vi "LDA2_Safety.vi"(1 "Adam Loop Count":i32, 2 "Ch Names":string[](array[string]), 3 "Values":dbl[](array[numeric]) format="%.2f") -> (0 "Scan comment":string)   [LabVIEW 2010]
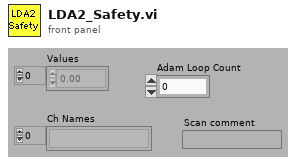
[diagram p1: front panel]
types:
  T1 = typedef "LVDateTimeRec.ctl" = cluster{"fractional second":dbl, "second":i32, "minute":i32, "hour":i32, "day of month":i32, "month":i32, "year":i32, "day of week":i32, "day of year":i32, "DST":i32}
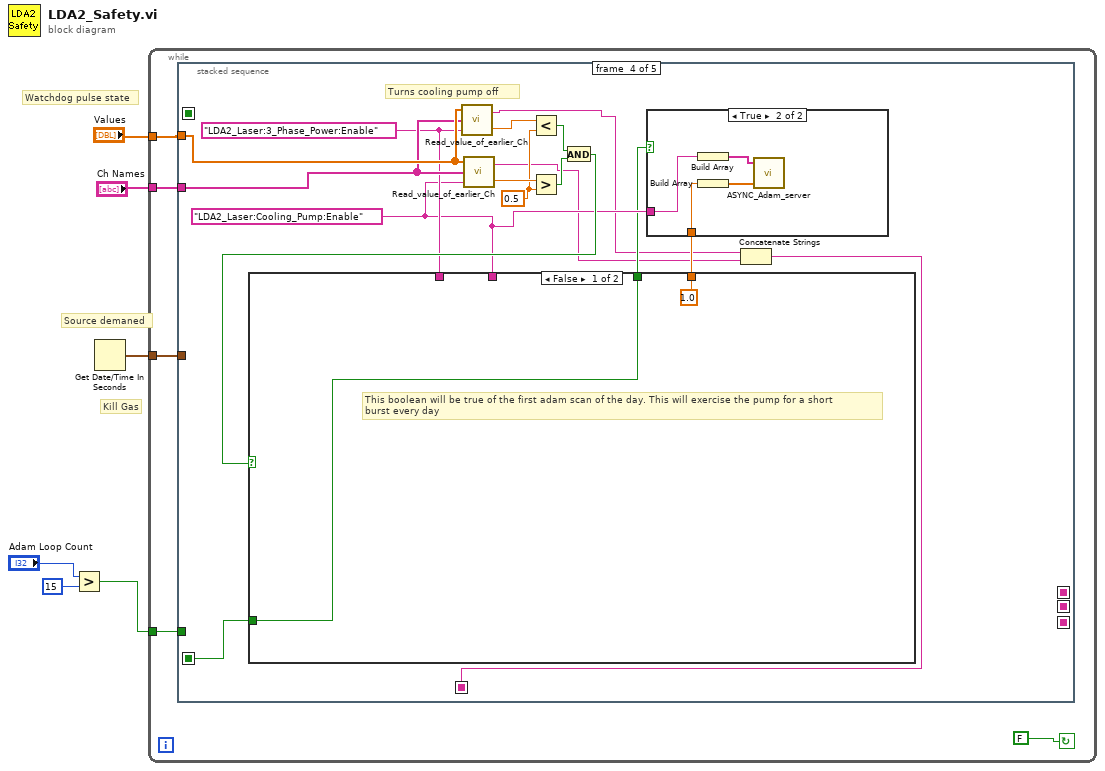
[diagram p0: block diagram]
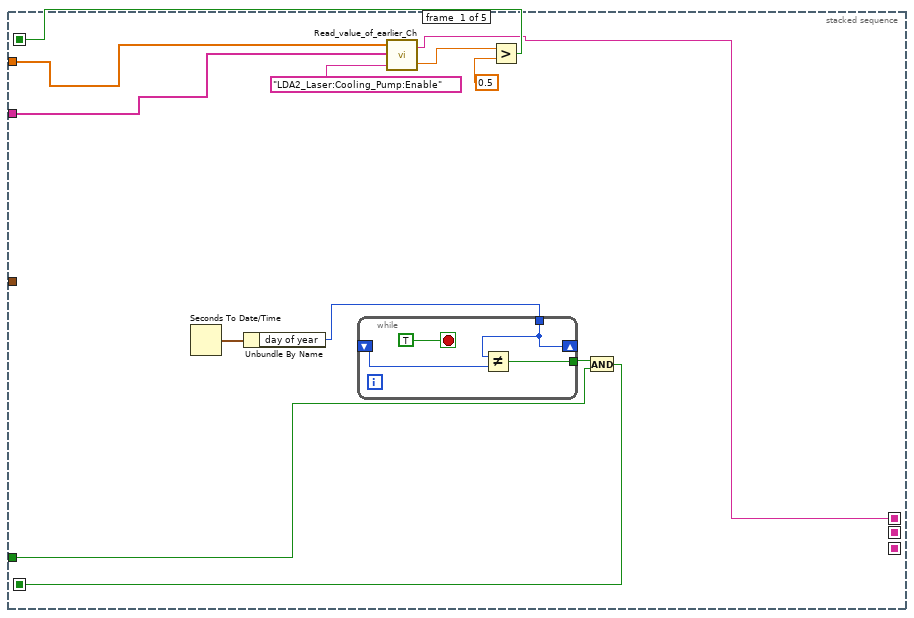
[diagram p2: hidden frame]
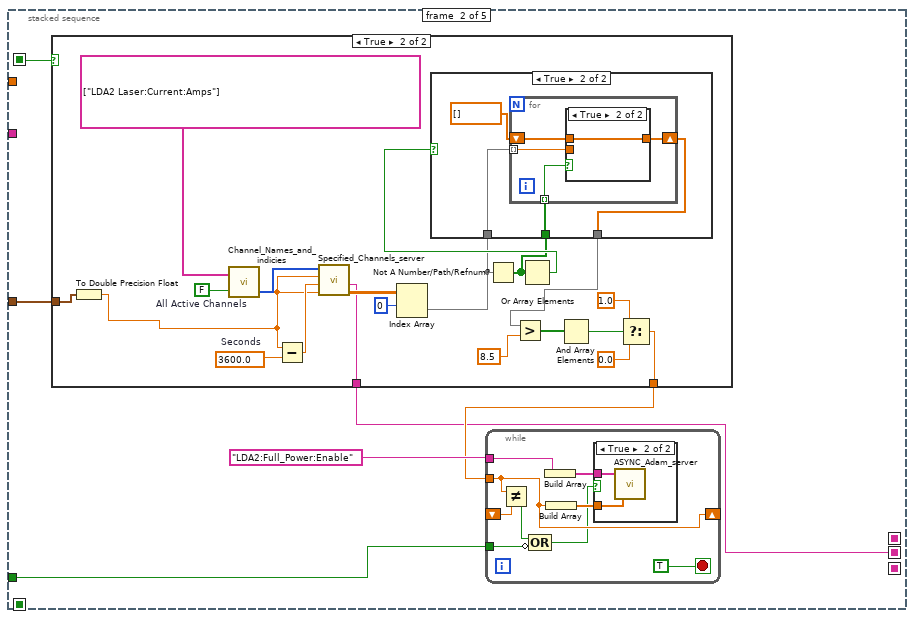
[diagram p3: hidden frame]
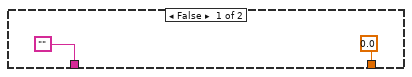
[diagram p5: hidden frame]
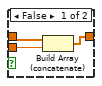
[diagram p7: hidden frame]
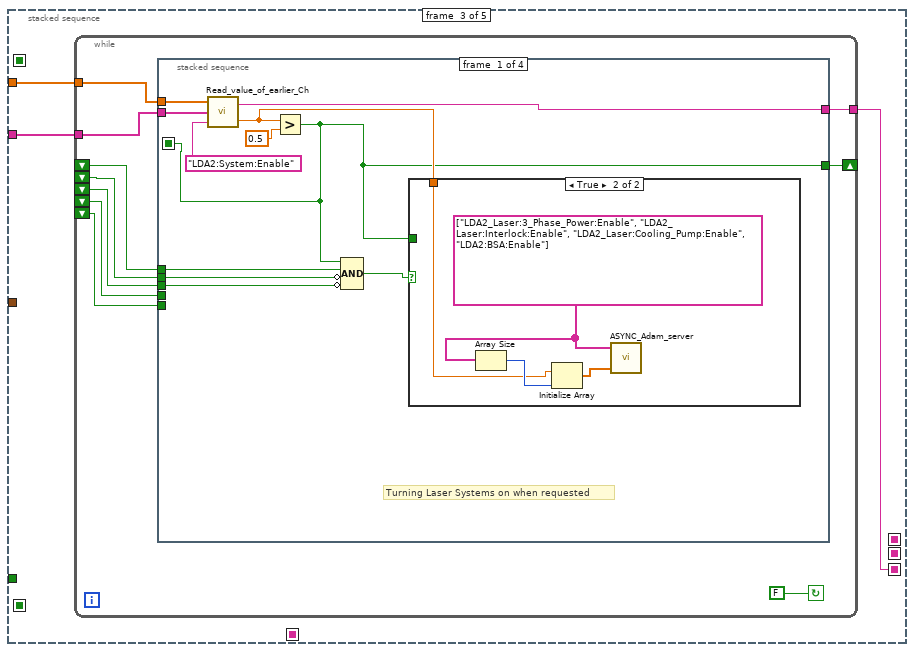
[diagram p8: hidden frame]
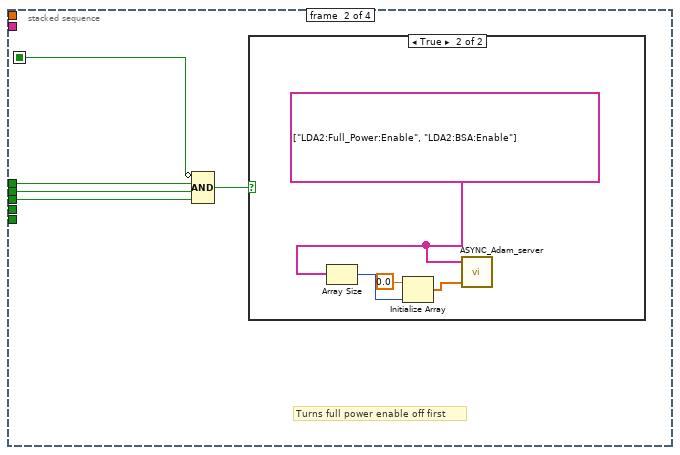
[diagram p10: hidden frame]
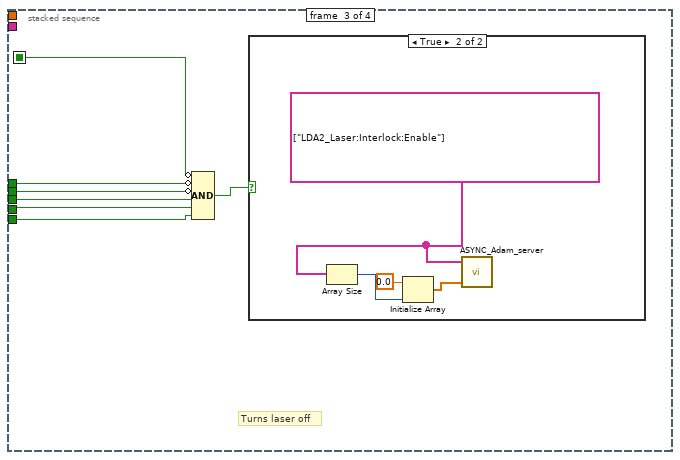
[diagram p12: hidden frame]
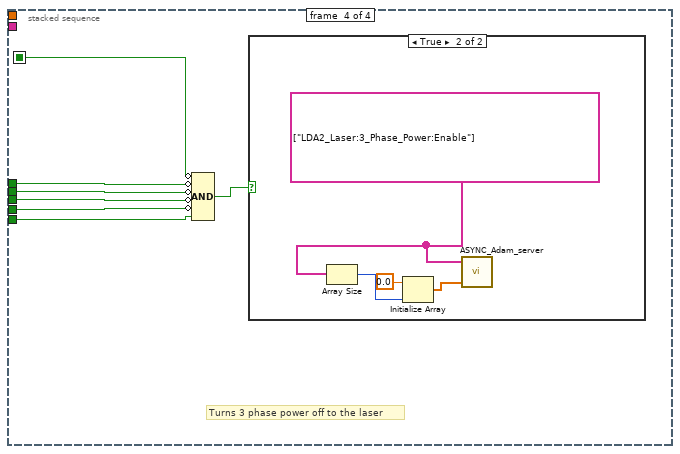
[diagram p14: hidden frame]
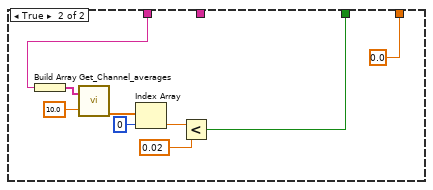
[diagram p17: hidden frame]
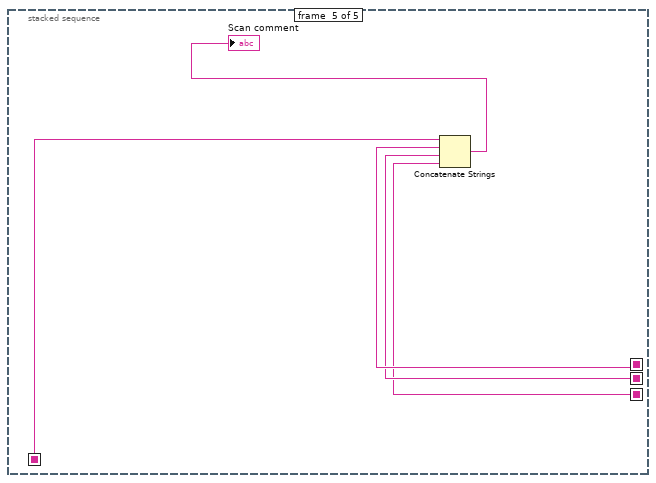
[diagram p18: hidden frame]
diagram:
  # "Source demaned"
  # "Watchdog pulse state"
  # "Kill Gas"
  n1 = Greater?(x="Adam Loop Count", y=15) -> (0:w2:bool)
  n2 = Get Date/Time In Seconds() -> (seconds since 1Jan1904=w1:timestamp)
  n3 = while {
    tunnel: "Ch Names" -> [w11]
    tunnel: "Values" -> [w10]
    tunnel: w2 -> [w8]
    tunnel: w1 -> [w7]
    stop <- FALSE continue-if-true
    n4 = stacked-sequence {
      seq-local: [w13 _ _ _ _] -> [_ _ _ w142 _]
      seq-local: [w21 _ _ _ _] -> [_ w32 _ _ _]
      seq-local: [w17 _ _ _ _] -> [_ _ _ _ w174]
      seq-local: [_ w28 _ _ _] -> [_ _ _ _ w173]
      seq-local: [_ _ w80 _ _] -> [_ _ _ _ w172]
      seq-local: [_ _ _ w139 _] -> [_ _ _ _ w170]
      tunnel: w11 -> [w22 _ w81 w152 _]
      tunnel: w10 -> [w23 _ w82 w153 _]
      tunnel: w8 -> [w12 w30 _ _ _]
      tunnel: w7 -> [_ w33 _ _ _]
      frame #0 {
        n5 = Seconds To Date/Time() -> (date time rec=w16:T1)  [unwired: 2 in]
        n6 = Unbundle By Name(w16) -> ("day of year"=w15:i32)
        n7 = while {
          shift-right: [w27] -> _
          shift-left: _ -> [w26]
          tunnel: w15 -> [w27]
          tunnel: [w25] -> w14
          stop <- TRUE stop-if-true
          n8 = Not Equal?(x=w27, y=w26) -> (x != y?=w25:bool)
        }
        n9 = call "Read_value_of_earlier_Ch.vi"("Desired Ch to Read"="LDA2_Laser:Cooling_Pump:Enable", "Ch names"=w22, "Present scan array"=w23) -> ("Value"=w19:dbl, "Scan comment"=w17:string)  [unwired: 1 in]
        n10 = Greater?(x=w19, y=0.5) -> (0:w21:bool)
        n11 = And(x=w14, y=w12) -> (x .and. y?=w13:bool)
      }
      frame #1 {
        n12 = case shown="True" w32 {
          tunnel: w33 -> [_ w66]
          tunnel: [0.0 ("y") w54] -> w29
          tunnel: ["" w48] -> w28
          frame False {
          }
          frame True {
            w64 = 3600.0  # Seconds
            w62 = FALSE  # All Active Channels
            n13 = To Double Precision Float(number=w66) -> (double precision float=w60:dbl)
            n14 = call "Channel_Names_and_indicies.vi"("All Active Channels"=w62, "Desired Ch Names"=string[] ["LDA2 Laser:Current:Amps"]) -> ("Indicies"=w63:i32[])  [unwired: 1 out]
            n15 = Subtract(x=w60, y=w64) -> (x-y=w65:dbl)
            n16 = call "Specified_Channels_server.vi"("End time"=w60, "Start time"=w65, "Clients time"=w60, "Requested channels"=w63) -> ("Output array"=w58:dbl[][], "Messages"=w48:string)  [unwired: 1 in, 3 out]
            n17 = Index Array(array=w58, index (row)=0) -> (element=w47:dbl[])  [unwired: 1 in]
            n18 = Not A Number/Path/Refnum?(number/path/refnum=w47) -> (NaN/Path/Refnum?=w50:bool[])
            n19 = Or Array Elements(Boolean array=w50) -> (logical OR=w51:bool)
            n20 = case shown="True" w51 {
              tunnel: w50 -> [_ w71]
              tunnel: w47 -> [w67 w70]
              tunnel: [w67 w68] -> w49
              frame False {
              }
              frame True {
                n21 = for {
                  shift-right: [w74] -> w68
                  shift-left: dbl[] [] -> [w73]
                  tunnel: w71 -> [w75] mode=indexing
                  tunnel: w70 -> [w72] mode=indexing
                  n22 = case shown="True" w75 {
                    tunnel: [w77 w79] -> w74
                    tunnel: w73 -> [w78 w79]
                    tunnel: w72 -> [w76 _]
                    frame False {
                      n23 = Build Array (concatenate)(w78, w76) -> (w77:dbl[])
                    }
                    frame True {
                    }
                  }
                }
              }
            }
            n24 = Greater?(x=w49, y=8.5) -> (0:w53:bool[])
            n25 = And Array Elements(Boolean array=w53) -> (logical AND=w52:bool)
            n26 = Select(t=1.0 ("y"), s=w52, f=0.0 ("y")) -> (s? t:f=w54:dbl)
          }
        }
        n27 = while {
          shift-right: [w38] -> _
          shift-left: _ -> [w39]
          tunnel: w29 -> [w38]
          tunnel: "LDA2:Full_Power:Enable" -> [w40]
          tunnel: w30 -> [w35]
          stop <- TRUE stop-if-true
          n28 = Not Equal?(x=w38, y=w39) -> (x != y?=w36:bool)
          n29 = Compound Arithmetic op=OR(w36, invert w35) -> (w34:bool)
          n30 = Build Array(w40) -> (w41:string[])
          n31 = Build Array(w38) -> (w42:dbl[])
          n32 = case shown="True" w34 {
            tunnel: w42 -> [_ w44]
            tunnel: w41 -> [_ w43]
            frame False {
            }
            frame True {
              n33 = call "ASYNC_Adam_server.vi"("Values"=w44, "Channel Names"=w43) -> ()  [unwired: 1 in, 3 out]
            }
          }
        }
      }
      frame #2 {
        n34 = while {
          tunnel: w82 -> [w92]
          tunnel: w81 -> [w91]
          shift-right: [w86] -> _
          shift-left: _ -> [w89]
          shift-left: _ -> [w88]
          shift-left: _ -> [w87]
          tunnel: [w85] -> w80
          shift-left: _ -> [w84]
          shift-left: _ -> [w83]
          stop <- FALSE continue-if-true
          n35 = stacked-sequence {
            seq-local: [w94 _ _ _] -> [_ w109 w120 w131]
            tunnel: w92 -> [w103 _ _ _]
            tunnel: w91 -> [w102 _ _ _]
            tunnel: w89 -> [w98 w112 w123 w134]
            tunnel: w88 -> [w97 w111 w122 w133]
            tunnel: w87 -> [w96 w110 w121 w132]
            tunnel: [w94 _ _ _] -> w86
            tunnel: [w95 _ _ _] -> w85
            tunnel: w84 -> [_ _ w118 w129]
            tunnel: w83 -> [_ _ w117 w128]
            frame #0 {
              # "Turning Laser Systems on when requested"
              n36 = call "Read_value_of_earlier_Ch.vi"("Desired Ch to Read"="LDA2:System:Enable", "Ch names"=w102, "Present scan array"=w103) -> ("Value"=w99:dbl, "Scan comment"=w95:string)  [unwired: 1 in]
              n37 = Greater?(x=w99, y=0.5) -> (0:w94:bool)
              n38 = Compound Arithmetic op=AND(w94, w98, invert w97, invert w96) -> (w93:bool)
              n39 = case shown="True" w93 {
                tunnel: w99 -> [_ w104]
                tunnel: w94 -> [_ _]
                frame False {
                }
                frame True {
                  w107 = string[] ["LDA2_Laser:3_Phase_Power:Enable", "LDA2_Laser:Interlock:Enable", "LDA2_Laser:Cooling_Pump:Enable", "LDA2:BSA:Enable"] ("Channel Names")
                  n40 = Array Size(array=w107) -> (size(s)=w105:i32)
                  n41 = Initialize Array(w104, w105) -> (w106:dbl[])
                  n42 = call "ASYNC_Adam_server.vi"("Values"=w106, "Channel Names"=w107) -> ()  [unwired: 1 in, 3 out]
                }
              }
            }
            frame #1 {
              # "Turns full power enable off first"
              n43 = Compound Arithmetic op=AND(invert w109, w112, w111, w110) -> (w108:bool)
              n44 = case shown="True" w108 {
                frame False {
                }
                frame True {
                  w113 = string[] ["LDA2:Full_Power:Enable", "LDA2:BSA:Enable"] ("Channel Names")
                  n45 = Array Size(array=w113) -> (size(s)=w115:i32)
                  n46 = Initialize Array(0.0, w115) -> (w116:dbl[])
                  n47 = call "ASYNC_Adam_server.vi"("Values"=w116, "Channel Names"=w113) -> ()  [unwired: 1 in, 3 out]
                }
              }
            }
            frame #2 {
              # "Turns laser off"
              n48 = Compound Arithmetic op=AND(invert w120, invert w123, invert w122, w121, w118, w117) -> (w119:bool)
              n49 = case shown="True" w119 {
                frame False {
                }
                frame True {
                  w124 = string[] ["LDA2_Laser:Interlock:Enable"] ("Channel Names")
                  n50 = Array Size(array=w124) -> (size(s)=w126:i32)
                  n51 = Initialize Array(0.0, w126) -> (w127:dbl[])
                  n52 = call "ASYNC_Adam_server.vi"("Values"=w127, "Channel Names"=w124) -> ()  [unwired: 1 in, 3 out]
                }
              }
            }
            frame #3 {
              # "Turns 3 phase power off to the laser"
              n53 = Compound Arithmetic op=AND(invert w131, invert w134, invert w133, invert w132, invert w129, w128) -> (w130:bool)
              n54 = case shown="True" w130 {
                frame False {
                }
                frame True {
                  w135 = string[] ["LDA2_Laser:3_Phase_Power:Enable"] ("Channel Names")
                  n55 = Array Size(array=w135) -> (size(s)=w137:i32)
                  n56 = Initialize Array(0.0, w137) -> (w138:dbl[])
                  n57 = call "ASYNC_Adam_server.vi"("Values"=w138, "Channel Names"=w135) -> ()  [unwired: 1 in, 3 out]
                }
              }
            }
          }
        }
      }
      frame #3 {
        w146 = "LDA2_Laser:3_Phase_Power:Enable" ("Desired Ch to Read")
        w151 = 0.5 ("y")
        w145 = "LDA2_Laser:Cooling_Pump:Enable" ("Desired Ch to Read")
        # "Turns cooling pump off"
        n58 = call "Read_value_of_earlier_Ch.vi"("Desired Ch to Read"=w146, "Ch names"=w152, "Present scan array"=w153) -> ("Value"=w150:dbl, "Scan comment"=w141:string)  [unwired: 1 in]
        n59 = call "Read_value_of_earlier_Ch.vi"("Desired Ch to Read"=w145, "Ch names"=w152, "Present scan array"=w153) -> ("Value"=w154:dbl, "Scan comment"=w140:string)  [unwired: 1 in]
        n60 = Less?(x=w150, y=w151) -> (x < y?=w149:bool)
        n61 = Greater?(x=w154, y=w151) -> (0:w148:bool)
        n62 = And(x=w149, y=w148) -> (x .and. y?=w147:bool)
        n63 = case shown="False" w147 {
          tunnel: w146 -> [_ w163]
          tunnel: w145 -> [_ _]
          tunnel: [w159 w162] -> w144
          tunnel: [1.0 ("element") 0.0 ("element")] -> w143
          tunnel: w142 -> [w159 _]
          frame False {
            # "This boolean will be true of the first adam scan of the day. This will exercise the pump for a short\nburst every day"
          }
          frame True {
            n64 = Build Array(w163) -> (w168:string[])
            n65 = call "Get_Channel_averages.vi"("Desired Ch Names"=w168, "Averaging time (mins)"=10.0) -> ("number"=w167:dbl[])  [unwired: 1 in, 2 out]
            n66 = Index Array(array=w167, index=0) -> (element=w165:dbl)
            n67 = Less?(x=w165, y=0.02) -> (x < y?=w162:bool)
          }
        }
        n68 = case shown="True" w144 {
          tunnel: w145 -> [_ w156]
          tunnel: w143 -> [_ w155]
          frame False {
          }
          frame True {
            n69 = Build Array(w156) -> (w157:string[])
            n70 = Build Array(w155) -> (w158:dbl[])
            n71 = call "ASYNC_Adam_server.vi"("Values"=w158, "Channel Names"=w157) -> ()  [unwired: 1 in, 3 out]
          }
        }
        n72 = Concatenate Strings(w141, w140) -> (w139:string)
      }
      frame #4 {
        n73 = Concatenate Strings(w170, w174, w173, w172) -> (→"Scan comment":string)
      }
    }
  }
